vi "Main.vi"() -> ()   [LabVIEW 2019]
panel:
  in  "Update":bool
  in  "Element to Update":enum16{"<None>", "Name", "Age", "Is Married?"}(ring)=enum."Age"
  in  "Stop":bool
  out "Current Customer Data":T1={"Name"="Adam", "Age"=23, "Is Married?"=TRUE, "Number of Updates"=8}
  in  "Is Married?":bool
  in  "Age":u8=23
  in  "Name":string="Adam"
  # "Data to Update"
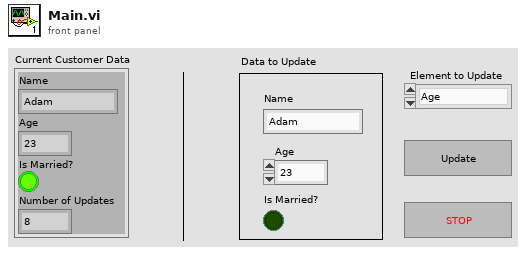
[diagram p1: front panel]
types:
  T1 = cluster{"Name":string, "Age":u8, "Is Married?":bool, "Number of Updates":i32}
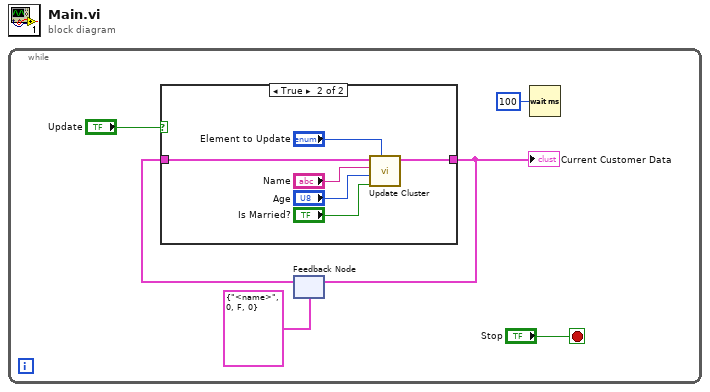
[diagram p0: block diagram]
diagram:
  n1 = while {
    stop <- "Stop" stop-if-true
    n2 = feedback #1(T1 {"Name"="<name>", "Age"=0, "Is Married?"=FALSE, "Number of Updates"=0} ("Current Customer Data")) -> (w2:T1)
    n3 = case shown="True" "Update" {
      tunnel: [w7 w9] -> w3
      tunnel: w2 -> [w7 w8]
      frame False {
      }
      frame True {
        n4 = call "Update Cluster.vi"("Element to Update"="Element to Update", "Is Married?"="Is Married?", "Age"="Age", "Name"="Name", "Customer Data in"=w8) -> ("Customer Data out"=w9:T1)  [unwired: 6 in]
      }
    }
    "Current Customer Data" <- w3
    n5 = feedback-in #1(w3) -> ()
    n6 = Wait (ms)(milliseconds to wait=u32 100) -> ()  [unwired: 1 out]
  }
